vi "Quadrature Continuous.vi"() -> ()   [LabVIEW 8.6]
uses:
  vi.lib/UeiDaq/UeiDaqCreateQuadEncoderSession.vi
  <libdir>/resource/objmgr/UeiDaq.rc
  vi.lib/UeiDaq/UeiDaqReadCounterDataUInt32.vi
  vi.lib/UeiDaq/UeiDaqConfigureTimingForBufferedO.vi
panel:
  in  "Samples per channel":i32
  in  "Sampling Rate (count/s)":dbl
  in  "Zero Index Phase":i32(ring) items=["Z high", "A low B low", "A low B high", "A high B low", "A high B high"]
  in  "Enable Zero Indexing":bool
  in  "Decoding Type":i32(ring) items=["1x", "2x", "4x"]
  out "Serial Number":string
  out "Name":string
  out "Encoder position":i32[][](array[numeric])
  in  "CI  Resource":string
  out "Total events acquired":u32
  in  "stop":bool
  # "Simulated Encoder (QUAD-604+dongle)"
  # "The resource string uses the following format:\n<deviceclass>://<IP Address>/Dev<DeviceId>/<Subsystem><ChannelList>\nex: simu://Dev0/Ai0:7 OR pdna://192.168.0.65/Dev1/Ao1,3"
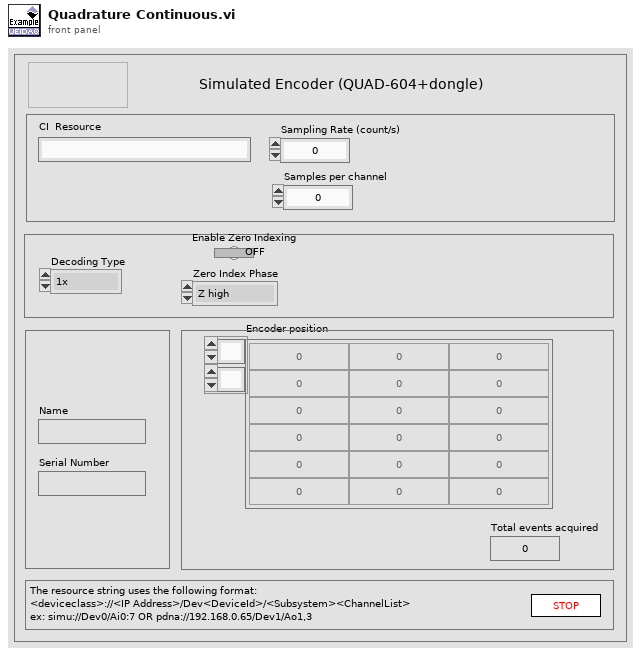
[diagram p1: front panel]
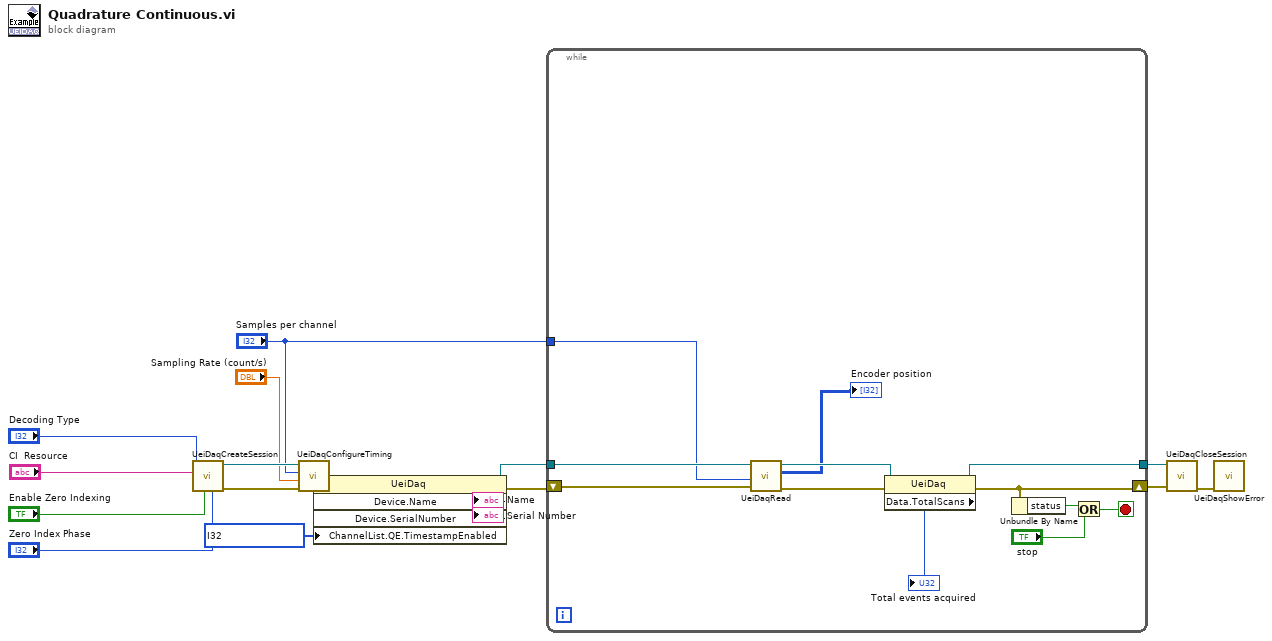
[diagram p0: block diagram]
diagram:
  w1 = i32[] ? items=["Disabled", "Enabled"] ("Channel List:Quadrature Encoder:The timestamp state")
  n1 = call-poly "UeiDaqCreateSession.vi"("Zero Index Phase"="Zero Index Phase", "Enable Zero Indexing"="Enable Zero Indexing", "Decoding Type"="Decoding Type", "Resource"="CI  Resource") -> ("error out"=w16:errorcluster, "UeiDaq Refnum Out"=w17:refnum<k20>)  [unwired: 4 in, 2 out]
  n2 = call-poly "UeiDaqConfigureTiming.vi"("error in (no error)"=w16, "Sampling rate"="Sampling Rate (count/s)", "Number of samples \nper channel"="Samples per channel", "UeiDaq Refnum In"=w17) -> ("error out"=w14:errorcluster, "UeiDaq Refnum Out"=w13:refnum<k20>)  [unwired: 3 in, 3 out]
  n3 = property class="UeiDaq"(reference=w13, error in=w14, "ChannelList.QE.TimestampEnabled"=w1) -> (reference out=w12:refnum<k20>, error out=w4:errorcluster, "Device.Name"=→"Name":string, "Device.SerialNumber"=→"Serial Number":string)
  n4 = while {
    tunnel: w12 -> [w30]
    tunnel: [w28] -> w9
    shift-right: [w22] -> w8
    shift-left: w4 -> [w21]
    tunnel: "Samples per channel" -> [w19]
    stop <- w23 stop-if-true
    n5 = call-poly "UeiDaqRead.vi"("error in (no error)"=w21, "numScans"=w19, "UeiDaq Refnum In"=w30) -> ("error out"=w29:errorcluster, "Raw Data"=→"Encoder position":u32[][], "UeiDaq Refnum Out"=w27:refnum<k20>)  [unwired: 6 out]
    n6 = property class="UeiDaq"(reference=w27, error in=w29) -> (reference out=w28:refnum<k20>, error out=w22:errorcluster, "Data.TotalScans"=→"Total events acquired":u32)
    n7 = Unbundle By Name(w22) -> ("status"=w24:bool)
    n8 = Or(x=w24, y="stop") -> (x .or. y?=w23:bool)
  }
  n9 = call "UeiDaqCloseSession.vi"("error in (no error)"=w8, "UeiDaq Refnum In"=w9) -> ("error out"=w18:errorcluster)  [unwired: 1 in, 8 out]
  n10 = call "UeiDaqShowError.vi"("error in (no error)"=w18) -> ()  [unwired: 2 in, 9 out]
